vi "ShowLineState.vi"(8 "错误输入（无错误）":errorcluster, 10 "LineState":enum16{"LineOff", "FAIL", "PASS"}(ring), 11 "¾€ów î‘BÒýÓÃ":refnum<vi>) -> (0 "错误输出":errorcluster)   [LabVIEW 2012]
uses:
  LineStateLamp.ctl
  Dev_State_Color.ctl
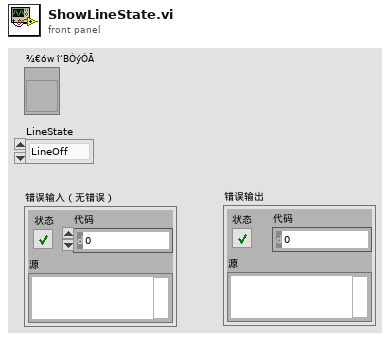
[diagram p1: front panel]
types:
  T1 = typedef "Dev_State_Color.ctl" = u32
  T2 = cluster{"DevState_Color":T1, "DevState_Color":T1}
  T3 = cluster{"DevState_Color":T1, "DevState_Color":T1}[]
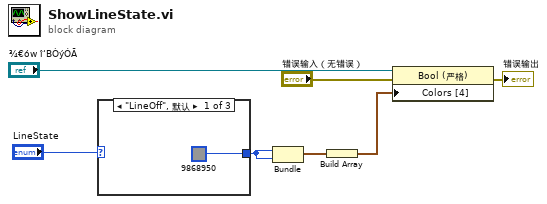
[diagram p0: block diagram]
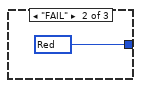
[diagram p2: hidden frame]
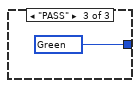
[diagram p3: hidden frame]
diagram:
  n1 = case shown="\"LineOff\", 默认" "LineState" {
    tunnel: [u32 9868950 w9 w10] -> w5
    frame "LineOff", Default {
    }
    frame "FAIL" {
      w9 = T1 16711680 items=["Yellow"=16772209, "Red"=16711680, "Green"=6618880] ("DevState_Color")
    }
    frame "PASS" {
      w10 = T1 6618880 items=["Yellow"=16772209, "Red"=16711680, "Green"=6618880] ("DevState_Color")
    }
  }
  n2 = Bundle("DevState_Color"=w5, "DevState_Color"=w5) -> (w4:T2)  [unwired: 1 in]
  n3 = Build Array(w4) -> (w3:T3)
  n4 = property class="Bool (严格)"(reference="¾€ów î‘BÒýÓÃ", error in="错误输入（无错误）", "Colors [4]"=w3) -> (error out=→"错误输出":errorcluster)  [unwired: 1 out]
